vi "Find Line Intersection.vi"(5 "Range":dbl=130.0, 7 "mm/pixel":dbl=0.4, 8 "picture":picture, 9 "Type":string, 11 "Color":string="Red") -> (0 "picture":picture, 1 "mm/pixel":dbl, 2 "Range":dbl, 3 "Result":cluster{"x":dbl, "y":dbl, "a":dbl})   [LabVIEW 2013]
uses:
  <vilib>/Analysis/NI_AALPro.lvlib
panel:
  out "G":u8[][](graph)
  out "B":u8[][](graph)
  out "R":u8[][](graph)
  in  "column":i32
  in  "row":i32
  in  "path to JPEG file":path
  in  "pixel center 2":cluster{"horizontal":i16, "vertical":i16}
  in  "pixel center":cluster{"horizontal":i16, "vertical":i16}
  in  "show?":bool=TRUE
  in  "Raw?":bool=TRUE
  # "Use these to calibrate a new color\nenable functions in block\ndiagram."
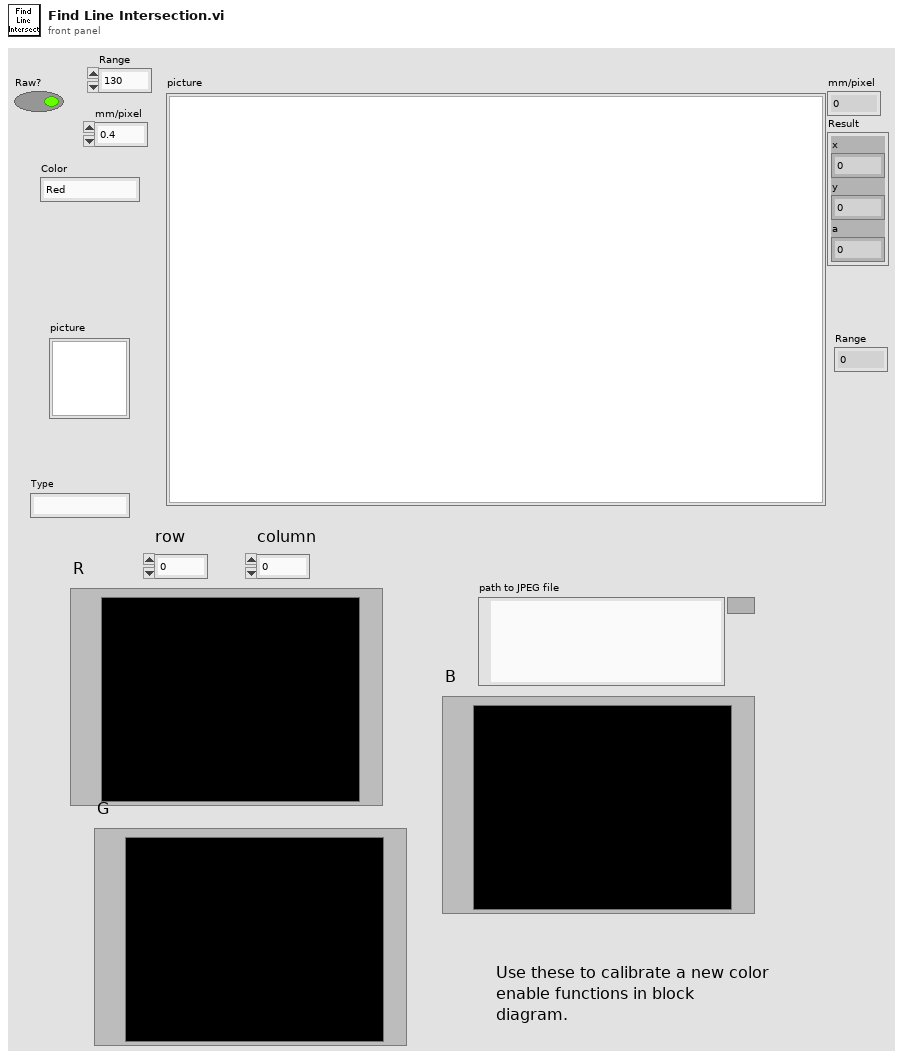
[diagram p1: front panel]
types:
  T1 = typedef "imagedata.ctl" = cluster{"image type":i32, "image depth":i32, "image":u8[], "mask":u8[], "colors":u32[], "Rectangle":cluster{"left":i16, "top":i16, "right":i16, "bottom":i16}}
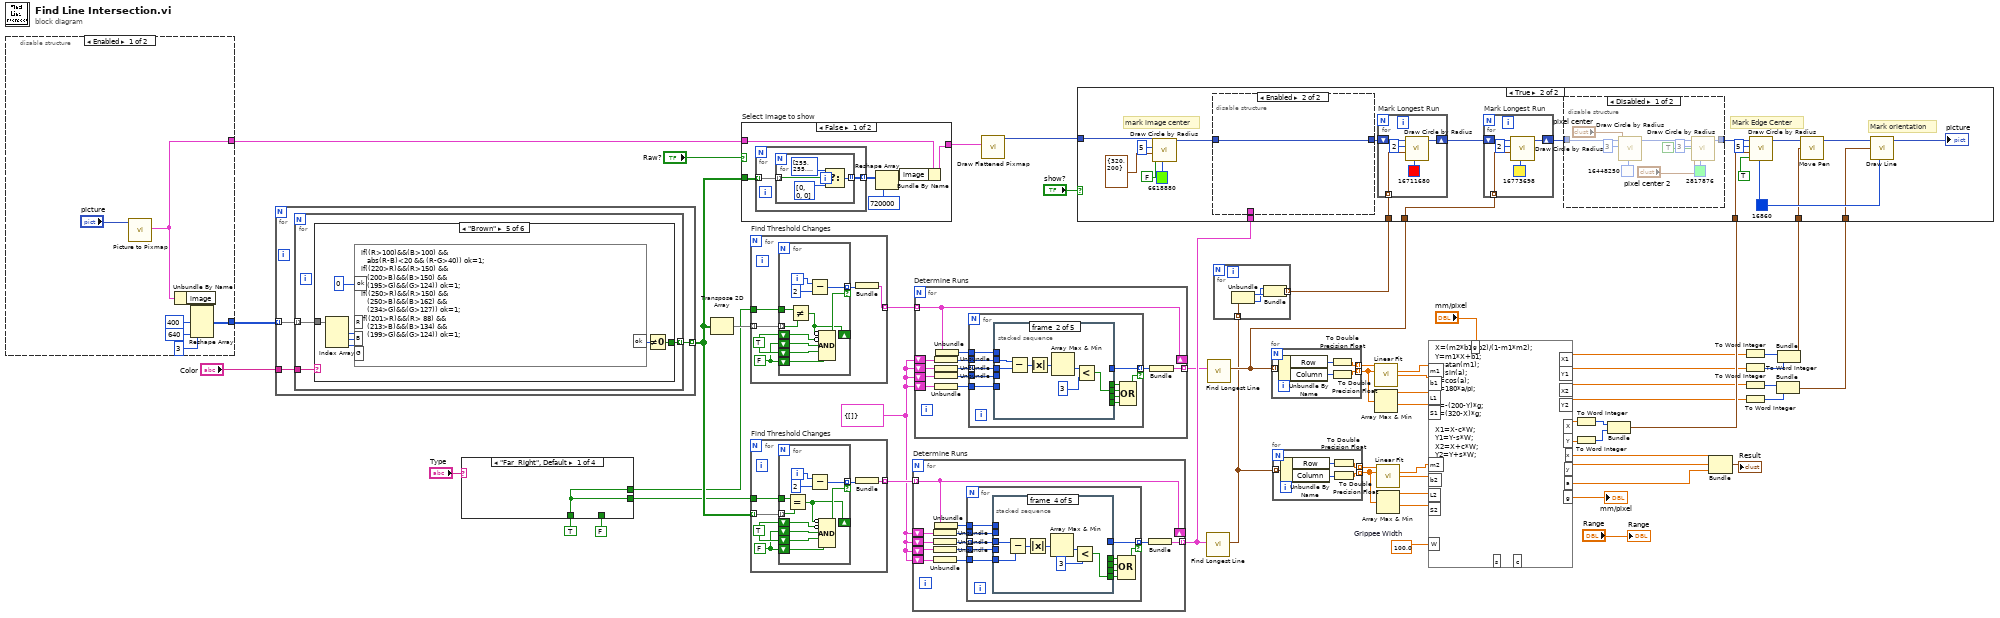
[diagram p0: block diagram]
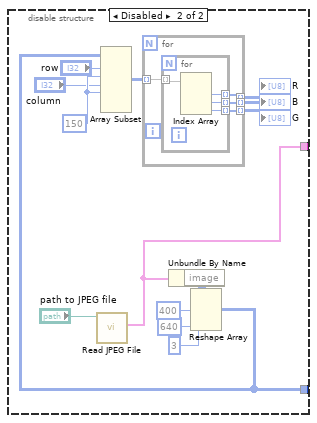
[diagram p5: hidden frame]
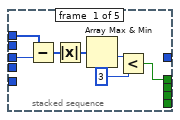
[diagram p6: hidden frame]
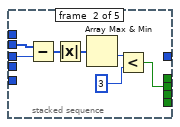
[diagram p7: hidden frame]
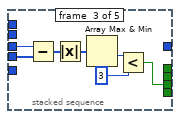
[diagram p8: hidden frame]
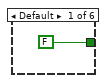
[diagram p11: hidden frame]
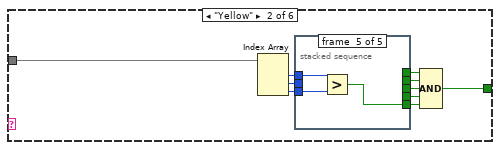
[diagram p12: hidden frame]
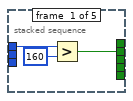
[diagram p13: hidden frame]
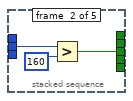
[diagram p14: hidden frame]
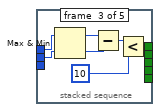
[diagram p15: hidden frame]
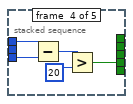
[diagram p16: hidden frame]
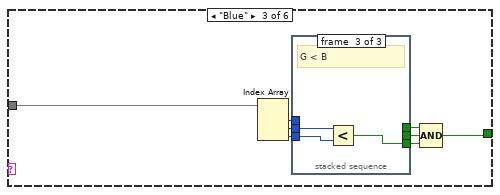
[diagram p17: hidden frame]
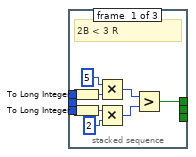
[diagram p18: hidden frame]
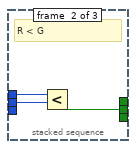
[diagram p19: hidden frame]
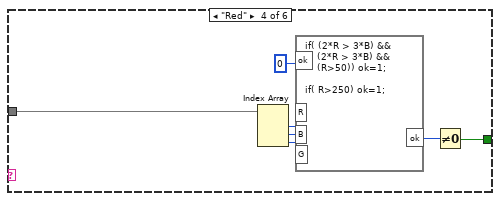
[diagram p20: hidden frame]
diagram:
  w24 = 100.0  # Grippee Width
  w41 = cluster{i32[]} {[]}
  n1 = disable-structure shown="Enabled" {
    disable-tunnel: [w60 w65] -> w2
    disable-tunnel: [w58 w66] -> w1
    frame Enabled {
      n2 = call <vilib>:"Picture to Pixmap.vi"("picture"="picture") -> ("image data"=w58:T1)  [unwired: 9 in, 1 out]
      n3 = Unbundle By Name(w58) -> ("image"=w59:u8[])
      n4 = Reshape Array(w59, 400 ("dimension size"), 640 ("dimension size"), 3 ("dimension size")) -> (w60:u8[][][])
    }
    frame Disabled {
      w73 = 150 ("length")
      n5 = call <vilib>:"Read JPEG File.vi"("path to JPEG file"="path to JPEG file") -> ("image data"=w66:T1)  [unwired: 8 in, 2 out]
      n6 = Unbundle By Name(w66) -> ("image"=w67:u8[])
      n7 = Reshape Array(w67, 400 ("dimension size"), 640 ("dimension size"), 3 ("dimension size")) -> (w65:u8[][][])
      n8 = Array Subset(array=w65, index (dim 0)="row", length (dim 0)=w73, index (dim 1)="column", length (dim 1)=w73) -> (w74:u8[][][])  [unwired: 2 in]
      n9 = for {
        tunnel: w74 -> [w82] mode=indexing
        tunnel: [w81] -> w75 mode=indexing
        tunnel: [w80] -> w76 mode=indexing
        tunnel: [w79] -> w77 mode=indexing
        n10 = for {
          tunnel: w82 -> [w86] mode=indexing
          tunnel: [w85] -> w81 mode=indexing
          tunnel: [w84] -> w80 mode=indexing
          tunnel: [w83] -> w79 mode=indexing
          n11 = Index Array(array=w86) -> (element #1=w85:u8, element #2=w84:u8, element #3=w83:u8)  [unwired: 3 in]
        }
      }
      "R" <- w75
      "B" <- w76
      "G" <- w77
    }
  }
  n12 = for {
    tunnel: w2 -> [w89] mode=indexing
    tunnel: [w88] -> w43 mode=indexing
    tunnel: "Color" -> [w87]
    n13 = for {
      tunnel: w89 -> [w92] mode=indexing
      tunnel: [w91] -> w88 mode=indexing
      tunnel: w87 -> [w90]
      n14 = case shown="\"Brown\"" w90 {
        tunnel: w92 -> [_ w103 w132 w154 w161 w168]
        tunnel: [FALSE w94 w125 w150 w157 w164] -> w91
        frame Default {
        }
        frame "Yellow" {
          n15 = Index Array(array=w103) -> (element #1=w102:u8, element #2=w101:u8, element #3=w100:u8)  [unwired: 3 in]
          n16 = stacked-sequence {
            tunnel: w102 -> [w106 _ w115 w118 w123]
            tunnel: w101 -> [_ w108 w116 _ _]
            tunnel: w100 -> [_ _ _ w119 w124]
            tunnel: [_ _ _ w120 _] -> w99
            tunnel: [w104 _ _ _ _] -> w98
            tunnel: [_ w107 _ _ _] -> w97
            tunnel: [_ _ w110 _ _] -> w96
            tunnel: [_ _ _ _ w122] -> w95
            frame #0 {
              n17 = Greater?(x=w106, y=u8 160) -> (0:w104:bool)
            }
            frame #1 {
              n18 = Greater?(x=w108, y=u8 160) -> (0:w107:bool)
            }
            frame #2 {
              n19 = Max & Min(x=w115, y=w116) -> (max(x,y)=w114:u8, min(x,y)=w113:u8)
              n20 = Subtract(x=w114, y=w113) -> (x-y=w112:u8)
              n21 = Less?(x=w112, y=u8 10) -> (x < y?=w110:bool)
            }
            frame #3 {
              n22 = Subtract(x=w118, y=w119) -> (x-y=w117:u8)
              n23 = Greater?(x=w117, y=u8 20) -> (0:w120:bool)
            }
            frame #4 {
              n24 = Greater?(x=w123, y=w124) -> (0:w122:bool)
            }
          }
          n25 = Compound Arithmetic op=AND(w96, w98, w97, w99, w95) -> (w94:bool)
        }
        frame "Blue" {
          n26 = Index Array(array=w132) -> (element #1=w131:u8, element #2=w130:u8, element #3=w129:u8)  [unwired: 3 in]
          n27 = stacked-sequence {
            tunnel: w131 -> [w137 w143 _]
            tunnel: w130 -> [_ w144 w147]
            tunnel: w129 -> [w141 _ w146]
            tunnel: [_ w142 _] -> w128
            tunnel: [_ _ w145] -> w127
            tunnel: [w138 _ _] -> w126
            frame #0 {
              # "2B < 3 R"
              n28 = To Long Integer(number=w137) -> (32bit integer=w134:i32)
              n29 = To Long Integer(number=w141) -> (32bit integer=w133:i32)
              n30 = Multiply(x=5, y=w134) -> (x*y=w136:i32)
              n31 = Multiply(x=w133, y=2) -> (x*y=w140:i32)
              n32 = Greater?(x=w136, y=w140) -> (0:w138:bool)
            }
            frame #1 {
              # "R < G"
              n33 = Less?(x=w143, y=w144) -> (x < y?=w142:bool)
            }
            frame #2 {
              # "G < B"
              n34 = Less?(x=w147, y=w146) -> (x < y?=w145:bool)
            }
          }
          n35 = Compound Arithmetic op=AND(w126, w128, w127) -> (w125:bool)
        }
        frame "Red" {
          n36 = Index Array(array=w154) -> (element #1=w153:u8, element #2=w152:u8, element #3=w151:u8)  [unwired: 3 in]
          n37 = formula code="if( (2*R > 3*B) &&\n    (2*R > 3*B) &&\n    (R>50)) ok=1; \n\nif( R>250) ok=1;"("R"=w153, "B"=w152, "G"=w151, "ok"=0) -> ("ok"=w148:i32)
          n38 = Not Equal To 0?(x=w148) -> (x != 0?=w150:bool)
        }
        frame "Brown" {
          n39 = Index Array(array=w161) -> (element #1=w160:u8, element #2=w159:u8, element #3=w158:u8)  [unwired: 3 in]
          n40 = formula code="if((R>100)&&(B>100) && \n   abs(R-B)<20 && (R-G>40)) ok=1; \nif((220>R)&&(R>150) &&\n   (200>B)&&(B>150) &&\n   (195>G)&&(G>124)) ok=1;\nif((250>R)&&(R>150) &&\n   (250>B)&&(B>162) &&\n   (234>G)&&(G>127)) ok=1;\nif((201>R)&&(R> 88) &&\n   (213>B)&&(B>134) &&\n   (199>G)&&(G>124)) ok=1;"("R"=w160, "B"=w159, "G"=w158, "ok"=0) -> ("ok"=w155:i32)
          n41 = Not Equal To 0?(x=w155) -> (x != 0?=w157:bool)
        }
        frame "Black" {
          n42 = Index Array(array=w168) -> (element #1=w167:u8, element #2=w166:u8, element #3=w165:u8)  [unwired: 3 in]
          n43 = formula code="if( (R<100) &&\n    (B<100) &&\n    (G<100)) ok=1;"("R"=w167, "B"=w166, "G"=w165, "ok"=0) -> ("ok"=w162:i32)
          n44 = Not Equal To 0?(x=w162) -> (x != 0?=w164:bool)
        }
      }
    }
  }
  n45 = case shown="\"Far_Right\", Default" "Type" {
    tunnel: FALSE -> [_ w171 w173 w174]
    tunnel: [w169 w171 w172 w174] -> w4
    tunnel: [w169 w170 w173 w174] -> w5
    tunnel: TRUE -> [w169 w170 w172 _]
    frame "Far_Right", Default {
    }
    frame "NR", "Near Right", "Near_Right" {
    }
    frame "FL", "Far Left", "Far_Left" {
    }
    frame "NL", "Near Left", "Near_Left" {
    }
  }
  n46 = Transpose 2D Array(2D array=w43) -> (transposed array=w56:bool[][])
  n47 = case "Select Image to show" shown="False" "Raw?" {
    tunnel: w1 -> [w180 w187]
    tunnel: [w176 w187] -> w44
    tunnel: w43 -> [w178 _]
    frame False {
      n48 = for {
        tunnel: w178 -> [w182] mode=indexing
        tunnel: [w181] -> w177 mode=indexing
        n49 = for {
          tunnel: w182 -> [w186] mode=indexing
          tunnel: [w183] -> w181 mode=indexing
          n50 = Select(t=u8[] [255, 255, 255], s=w186, f=u8[] [0, 0, 0]) -> (s? t:f=w183:u8[])
        }
      }
      n51 = Reshape Array(w177, 720000 ("dimension size")) -> (w179:u8[])
      n52 = Bundle By Name(cluster=w180, "image"=w179) -> (w176:T1)
    }
    frame True {
    }
  }
  n53 = for "Find Threshold Changes" {
    tunnel: w56 -> [w193] mode=indexing
    tunnel: [w189] -> w55 mode=indexing
    tunnel: w4 -> [w188]
    w191 = FALSE
    w192 = TRUE
    n54 = for {
      tunnel: w193 -> [w195] mode=indexing
      shift-right: [w196] -> _
      shift-left: w192 -> [w203]
      shift-left: w191 -> [w202]
      shift-left: w192 -> [w201]
      shift-left: w191 -> [w200]
      tunnel: [w199] -> w190 mode=indexing if=w198
      tunnel: w188 -> [w194]
      i -> [w204]
      n55 = Not Equal?(x=w194, y=w195) -> (x != y?=w196:bool)
      n56 = Subtract(x=w204, y=2) -> (x-y=w199:i32)
      n57 = Compound Arithmetic op=AND(invert w196, invert w203, w202, w201, w200) -> (w198:bool)
    }
    n58 = Bundle(w190) -> (w189:cluster{i32[]})  [unwired: 1 in]
  }
  n59 = for "Find Threshold Changes" {
    tunnel: w43 -> [w210] mode=indexing
    tunnel: [w206] -> w42 mode=indexing
    tunnel: w5 -> [w205]
    w208 = FALSE
    w209 = TRUE
    n60 = for {
      tunnel: w210 -> [w213] mode=indexing
      shift-right: [w212] -> _
      shift-left: w209 -> [w219]
      shift-left: w208 -> [w218]
      shift-left: w209 -> [w217]
      shift-left: w208 -> [w216]
      tunnel: [w215] -> w207 mode=indexing if=w214
      tunnel: w205 -> [w211]
      i -> [w221]
      n61 = Equal?(x=w211, y=w213) -> (x = y?=w212:bool)
      n62 = Subtract(x=w221, y=2) -> (x-y=w215:i32)
      n63 = Compound Arithmetic op=AND(invert w212, invert w219, w218, w217, w216) -> (w214:bool)
    }
    n64 = Bundle(w207) -> (w206:cluster{i32[]})  [unwired: 1 in]
  }
  n65 = for "Determine Runs" {
    tunnel: w42 -> [w232] mode=indexing
    shift-right: [w232] -> _
    shift-left: w41 -> [w231]
    shift-left: w41 -> [w233]
    shift-left: w41 -> [w230]
    shift-left: w41 -> [w229]
    tunnel: [w228] -> w39 mode=indexing
    n66 = Unbundle(w231) -> (w223:i32[])
    n67 = Unbundle(w233) -> (w224:i32[])
    n68 = Unbundle(w230) -> (w225:i32[])
    n69 = Unbundle(w229) -> (w226:i32[])
    n70 = Unbundle(w232) -> (w222:i32[])
    n71 = for {
      tunnel: w224 -> [w243] mode=indexing
      tunnel: w222 -> [w244]
      tunnel: w223 -> [w242]
      tunnel: w225 -> [w238]
      tunnel: w226 -> [w236]
      tunnel: [w235] -> w227 mode=indexing if=w234
      n72 = stacked-sequence {
        tunnel: w244 -> [w251 _ _ _ _]
        tunnel: w243 -> [w250 w258 w260 w268 w273]
        tunnel: w242 -> [_ w253 _ _ _]
        tunnel: [_ w252 _ _ _] -> w241
        tunnel: [w245 _ _ _ _] -> w240
        tunnel: [_ _ w261 _ _] -> w239
        tunnel: w238 -> [_ _ w259 _ _]
        tunnel: [_ _ _ w267 _] -> w237
        tunnel: w236 -> [_ _ _ w266 _]
        tunnel: [_ _ _ _ w273] -> w235
        frame #0 {
          n73 = Subtract(x=w251, y=w250) -> (x-y=w249:i32[])
          n74 = Absolute Value(x=w249) -> (abs(x)=w248:i32[])
          n75 = Array Max & Min(array=w248) -> (min value=w247:i32)  [unwired: 3 out]
          n76 = Less?(x=w247, y=3) -> (x < y?=w245:bool)
        }
        frame #1 {
          n77 = Subtract(x=w253, y=w258) -> (x-y=w257:i32[])
          n78 = Absolute Value(x=w257) -> (abs(x)=w256:i32[])
          n79 = Array Max & Min(array=w256) -> (min value=w255:i32)  [unwired: 3 out]
          n80 = Less?(x=w255, y=3) -> (x < y?=w252:bool)
        }
        frame #2 {
          n81 = Subtract(x=w260, y=w259) -> (x-y=w265:i32[])
          n82 = Absolute Value(x=w265) -> (abs(x)=w264:i32[])
          n83 = Array Max & Min(array=w264) -> (min value=w263:i32)  [unwired: 3 out]
          n84 = Less?(x=w263, y=3) -> (x < y?=w261:bool)
        }
        frame #3 {
          n85 = Subtract(x=w268, y=w266) -> (x-y=w272:i32[])
          n86 = Absolute Value(x=w272) -> (abs(x)=w271:i32[])
          n87 = Array Max & Min(array=w271) -> (min value=w270:i32)  [unwired: 3 out]
          n88 = Less?(x=w270, y=3) -> (x < y?=w267:bool)
        }
        frame #4 {
        }
      }
      n89 = Compound Arithmetic op=OR(w240, w241, w239, w237) -> (w234:bool)
    }
    n90 = Bundle(w227) -> (w228:cluster{i32[]})  [unwired: 1 in]
  }
  n91 = for "Determine Runs" {
    tunnel: w55 -> [w284] mode=indexing
    shift-right: [w284] -> _
    shift-left: w41 -> [w283]
    shift-left: w41 -> [w285]
    shift-left: w41 -> [w282]
    shift-left: w41 -> [w281]
    tunnel: [w280] -> w38 mode=indexing
    n92 = Unbundle(w283) -> (w275:i32[])
    n93 = Unbundle(w285) -> (w276:i32[])
    n94 = Unbundle(w282) -> (w277:i32[])
    n95 = Unbundle(w281) -> (w278:i32[])
    n96 = Unbundle(w284) -> (w274:i32[])
    n97 = for {
      tunnel: w276 -> [w295] mode=indexing
      tunnel: w274 -> [w296]
      tunnel: w275 -> [w294]
      tunnel: w277 -> [w290]
      tunnel: w278 -> [w288]
      tunnel: [w287] -> w279 mode=indexing if=w286
      n98 = stacked-sequence {
        tunnel: w296 -> [w303 _ _ _ _]
        tunnel: w295 -> [w302 w310 w312 w320 w325]
        tunnel: w294 -> [_ w305 _ _ _]
        tunnel: [_ w304 _ _ _] -> w293
        tunnel: [w297 _ _ _ _] -> w292
        tunnel: [_ _ w313 _ _] -> w291
        tunnel: w290 -> [_ _ w311 _ _]
        tunnel: [_ _ _ w319 _] -> w289
        tunnel: w288 -> [_ _ _ w318 _]
        tunnel: [_ _ _ _ w325] -> w287
        frame #0 {
          n99 = Subtract(x=w303, y=w302) -> (x-y=w301:i32[])
          n100 = Absolute Value(x=w301) -> (abs(x)=w300:i32[])
          n101 = Array Max & Min(array=w300) -> (min value=w299:i32)  [unwired: 3 out]
          n102 = Less?(x=w299, y=3) -> (x < y?=w297:bool)
        }
        frame #1 {
          n103 = Subtract(x=w305, y=w310) -> (x-y=w309:i32[])
          n104 = Absolute Value(x=w309) -> (abs(x)=w308:i32[])
          n105 = Array Max & Min(array=w308) -> (min value=w307:i32)  [unwired: 3 out]
          n106 = Less?(x=w307, y=3) -> (x < y?=w304:bool)
        }
        frame #2 {
          n107 = Subtract(x=w312, y=w311) -> (x-y=w317:i32[])
          n108 = Absolute Value(x=w317) -> (abs(x)=w316:i32[])
          n109 = Array Max & Min(array=w316) -> (min value=w315:i32)  [unwired: 3 out]
          n110 = Less?(x=w315, y=3) -> (x < y?=w313:bool)
        }
        frame #3 {
          n111 = Subtract(x=w320, y=w318) -> (x-y=w324:i32[])
          n112 = Absolute Value(x=w324) -> (abs(x)=w323:i32[])
          n113 = Array Max & Min(array=w323) -> (min value=w322:i32)  [unwired: 3 out]
          n114 = Less?(x=w322, y=3) -> (x < y?=w319:bool)
        }
        frame #4 {
        }
      }
      n115 = Compound Arithmetic op=OR(w292, w293, w291, w289) -> (w286:bool)
    }
    n116 = Bundle(w279) -> (w280:cluster{i32[]})  [unwired: 1 in]
  }
  n117 = call <vilib>:"Draw Flattened Pixmap.vi"("image data"=w44) -> ("new picture"=w57:picture)  [unwired: 8 in]
  n118 = call "Find Longest Line.vi"("Array"=w39) -> ("Edge"=w34:cluster{"Column":i32, "Row":i32}[])  [unwired: 10 in]
  n119 = call "Find Longest Line.vi"("Array"=w38) -> ("Edge"=w37:cluster{"Column":i32, "Row":i32}[])  [unwired: 10 in]
  n120 = for {
    tunnel: w34 -> [w329] mode=indexing
    tunnel: [w326] -> w40 mode=indexing
    n121 = Unbundle(w329) -> ("Column"=w328:i32, "Row"=w327:i32)
    n122 = Bundle("Row"=w327, "Column"=w328) -> (w326:cluster{"Row":i32, "Column":i32})  [unwired: 1 in]
  }
  n123 = for {
    tunnel: w37 -> [w332] mode=indexing
    tunnel: [w331] -> w48 mode=indexing
    tunnel: [w330] -> w46 mode=indexing
    n124 = Unbundle By Name(w332) -> ("Row"=w333:i32, "Column"=w334:i32)
    n125 = To Double Precision Float(number=w333) -> (double precision float=w331:dbl)
    n126 = To Double Precision Float(number=w334) -> (double precision float=w330:dbl)
  }
  n127 = for {
    tunnel: [w335] -> _ mode=indexing
    tunnel: [w337] -> w36 mode=indexing
    tunnel: [w336] -> w35 mode=indexing
    tunnel: w34 -> [w335] mode=indexing
    n128 = Unbundle By Name(w335) -> ("Row"=w338:i32, "Column"=w339:i32)
    n129 = To Double Precision Float(number=w338) -> (double precision float=w337:dbl)
    n130 = To Double Precision Float(number=w339) -> (double precision float=w336:dbl)
  }
  n131 = call <vilib>:"Linear Fit.vi"("Y"=w48, "X"=w46) -> ("slope"=w32:dbl, "intercept"=w33:dbl)  [unwired: 9 in, 3 out]
  n132 = Array Max & Min(array=w46) -> (max value=w27:dbl, min value=w26:dbl)  [unwired: 2 out]
  n133 = call <vilib>:"Linear Fit.vi"("Y"=w36, "X"=w35) -> ("slope"=w30:dbl, "intercept"=w31:dbl)  [unwired: 9 in, 3 out]
  n134 = Array Max & Min(array=w35) -> (max value=w29:dbl, min value=w28:dbl)  [unwired: 2 out]
  n135 = formula code="X=(m2*b1+b2)/(1-m1*m2);\nY=m1*X+b1;\na=atan(m1);\ns=sin(a);\nc=cos(a);\na=180*a/pi;\n\nx=-(200-Y)*g;\ny=(320-X)*g;\n\nX1=X-c*W;\nY1=Y-s*W;\nX2=X+c*W;\nY2=Y+s*W;"("m1"=w32, "b1"=w33, "b2"=w31, "m2"=w30, "L2"=w29, "S2"=w28, "L1"=w27, "S1"=w26, "W"=w24, "g"="mm/pixel") -> ("x"=w22:dbl, "y"=w23:dbl, "a"=w21:dbl, "g"=→"mm/pixel":dbl, "X"=w20:dbl, "Y"=w19:dbl, "X1"=w18:dbl, "Y1"=w17:dbl, "X2"=w14:dbl, "Y2"=w13:dbl)  [unwired: 2 out]
  n136 = To Word Integer(number=w19) -> (16bit integer=w50:i16)
  n137 = To Word Integer(number=w20) -> (16bit integer=w51:i16)
  n138 = Bundle(w51, w50) -> (w49:cluster{i16, i16})  [unwired: 1 in]
  n139 = Bundle("x"=w22, "y"=w23, "a"=w21) -> (→"Result":cluster{"x":dbl, "y":dbl, "a":dbl})  [unwired: 1 in]
  n140 = To Word Integer(number=w14) -> (16bit integer=w16:i16)
  n141 = To Word Integer(number=w13) -> (16bit integer=w15:i16)
  n142 = To Word Integer(number=w18) -> (16bit integer=w54:i16)
  n143 = To Word Integer(number=w17) -> (16bit integer=w53:i16)
  n144 = Bundle(w16, w15) -> (w12:cluster{i16, i16})  [unwired: 1 in]
  n145 = Bundle(w54, w53) -> (w52:cluster{i16, i16})  [unwired: 1 in]
  n146 = case shown="True" "show?" {
    tunnel: w57 -> [_ w361]
    tunnel: w39 -> [_ w356]
    tunnel: w52 -> [_ w343]
    tunnel: w49 -> [_ w349]
    tunnel: w40 -> [_ w348]
    tunnel: w37 -> [_ w345]
    tunnel: w12 -> [_ w342]
    frame False {
    }
    frame True {
      w347 = u32 16860
      # "Mark orientation"
      # "Mark Edge Center"
      # "mark image center"
      n147 = call <vilib>:"Draw Circle by Radius.vi"("color(black)"=u32 6618880, "fill?(F)"=FALSE, "pixel center"=cluster{"horizontal":i16, "vertical":i16} {"horizontal"=320, "vertical"=200}, "radius"=i16 5, "picture"=w361) -> ("new picture"=w355:picture)  [unwired: 6 in]
      n148 = disable-structure shown="Enabled" {
        disable-tunnel: w356 -> [w375 _]
        disable-tunnel: w355 -> [w374 w388]
        disable-tunnel: [w373 w388] -> w354
        frame Disabled {
          n149 = for "Mark Runs" {
            shift-right: [w379] -> w373
            shift-left: w374 -> [w380]
            tunnel: w375 -> [w378] mode=indexing
            i -> [w376]
            n150 = Unbundle(w378) -> (w377:i32[])
            n151 = for {
              tunnel: w377 -> [w384] mode=indexing
              shift-right: [w386] -> w379
              shift-left: w380 -> [w387]
              tunnel: w376 -> [w381]
              n152 = Bundle(w384, w381) -> (w383:cluster{i32, i32})  [unwired: 1 in]
              n153 = call <vilib>:"Draw Circle by Radius.vi"("color(black)"=u32 9567230, "pixel center"=w383, "radius"=i16 2, "picture"=w387) -> ("new picture"=w386:picture)  [unwired: 7 in]
            }
          }
        }
        frame Enabled {
        }
      }
      n154 = for "Mark Longest Run" {
        shift-right: [w397] -> w346
        shift-left: w354 -> [w398]
        tunnel: w348 -> [w394] mode=indexing
        n155 = call <vilib>:"Draw Circle by Radius.vi"("color(black)"=u32 16711680, "pixel center"=w394, "radius"=i16 2, "picture"=w398) -> ("new picture"=w397:picture)  [unwired: 7 in]
      }
      n156 = for "Mark Longest Run" {
        shift-right: [w392] -> w341
        shift-left: w346 -> [w393]
        tunnel: w345 -> [w389] mode=indexing
        n157 = call <vilib>:"Draw Circle by Radius.vi"("color(black)"=u32 16773698, "pixel center"=w389, "radius"=i16 2, "picture"=w393) -> ("new picture"=w392:picture)  [unwired: 7 in]
      }
      n158 = disable-structure shown="Disabled" {
        disable-tunnel: w341 -> [w370 w372]
        disable-tunnel: [w364 w372] -> w340
        frame Disabled {
          n159 = call <vilib>:"Draw Circle by Radius.vi"("color(black)"=u32 16448250, "pixel center"="pixel center", "radius"=i16 3, "picture"=w370) -> ("new picture"=w365:picture)  [unwired: 7 in]
          n160 = call <vilib>:"Draw Circle by Radius.vi"("color(black)"=u32 2817876, "fill?(F)"=TRUE, "pixel center"="pixel center 2", "radius"=i16 3, "picture"=w365) -> ("new picture"=w364:picture)  [unwired: 6 in]
        }
        frame Enabled {
        }
      }
      n161 = call <vilib>:"Draw Circle by Radius.vi"("color(black)"=w347, "fill?(F)"=TRUE, "pixel center"=w349, "radius"=i16 5, "picture"=w340) -> ("new picture"=w351:picture)  [unwired: 6 in]
      n162 = call <vilib>:"Move Pen.vi"("new position"=w343, "picture"=w351) -> ("new picture"=w350:picture)  [unwired: 3 in]
      n163 = call <vilib>:"Draw Line.vi"("picture"=w350, "end point"=w342, "color(black)"=w347) -> ("new picture"=→"picture":picture)  [unwired: 6 in]
    }
  }
  "Range" <- "Range"
